vi "reward_behavior_timeout_10s_probes.vi"() -> ()   [LabVIEW 2019]
doc: "The myRIO Project template acquires acceleration data from the onboard accelerometer and displays the changes of acceleration values in a waveform chart."
uses:
  <vilib>/Analysis/Matrix/Datatypes/RealMatrix.ctl
  <vilib>/myRIO/Common/Instrument Driver Framework/myRIO v1.0/Encoder/typedefs/Encoder Signal Mode.ctl
  <vilib>/myRIO/Instrument Drivers/Onboard IO/Encoder/typedefs/Encoder Reference.ctl
  <vilib>/myRIO/Common/Instrument Driver Framework/Utilities/typedefs/myRIO Generic Hardware Reference.ctl
  <vilib>/myRIO/Common/Instrument Driver Framework/Utilities/typedefs/Hardware Version Enum.ctl
  <vilib>/myRIO/Common/Instrument Driver Framework/Utilities/typedefs/myRIO v1.0 Reference.ctl
  <vilib>/myRIO/Common/Instrument Driver Framework/Utilities/typedefs/Generic FPGA Reference.ctl
  <vilib>/myRIO/Common/Instrument Driver Framework/myRIO v1.0/Encoder/typedefs/Encoder Channels Enum.ctl
  <vilib>/myRIO/Common/Instrument Driver Framework/myRIO v1.0/Encoder/typedefs/Encoder Configuration v1.0.ctl
  <vilib>/userdefined/High Color/nirio_resource_hc.ctl
  <vilib>/myRIO/Instrument Drivers/Onboard IO/DIO/typedefs/DIO Reference.ctl
  <vilib>/myRIO/Common/Instrument Driver Framework/myRIO v1.0/DIO/typedefs/DIO Channels List.ctl
  <vilib>/myRIO/Common/Instrument Driver Framework/myRIO v1.0/DIO/typedefs/DIO Channels Enum.ctl
  <vilib>/myRIO/Common/Instrument Driver Framework/Utilities/vis/Is FPGA Ref Available.vi
  <vilib>/myRIO/Common/Instrument Driver Framework/myRIO v1.0/Encoder/vis/myRIO v1.1 Open Encoder.vi
  <vilib>/myRIO/Instrument Drivers/Onboard IO/Encoder/vis/Read.vi
  <vilib>/myRIO/Common/Instrument Driver Framework/myRIO v1.0/DIO/vis/myRIO v1.1 Open DIO.vi
  <vilib>/myRIO/Instrument Drivers/Onboard IO/DIO/vis/Write.vi
  <vilib>/myRIO/Instrument Drivers/Onboard IO/DIO/vis/Read.vi
  <vilib>/myRIO/Common/Instrument Driver Framework/Utilities/vis/Validate Channels.vi
  <vilib>/myRIO/Common/Instrument Driver Framework/myRIO v1.0/Encoder/vis/myRIO v1.0 Reserve Encoder.vi
  <vilib>/myRIO/Common/Instrument Driver Framework/myRIO v1.0/DIO/vis/myRIO v1.0 Reserve DIO.vi
  <vilib>/myRIO/Common/Instrument Driver Framework/myRIO v1.0/Encoder/vis/myRIO v1.0 Build MUX Configuration Encoder.vi
  <vilib>/myRIO/Common/Instrument Driver Framework/myRIO v1.0/Resource Manager/vis/myRIO v1.0 Reserve Channel List.vi
  <vilib>/myRIO/Common/Instrument Driver Framework/myRIO v1.0/DIO/vis/myRIO v1.0 Build MUX Configuration DIO.vi
  <vilib>/myRIO/Common/Instrument Driver Framework/myRIO v1.0/Resource Manager/vis/myRIO v1.0 Create Configuration List.vi
  <vilib>/myRIO/Common/Instrument Driver Framework/myRIO v1.0/Resource Manager/vis/myRIO v1.0 Reserve Channel.vi
  <vilib>/myRIO/Common/Instrument Driver Framework/myRIO v1.0/Resource Manager/vis/myRIO v1.0 Unreserve Channel.vi
  <vilib>/myRIO/Common/Instrument Driver Framework/myRIO v1.0/Resource Manager/vis/myRIO v1.0 Build Mutex Name.vi
  <vilib>/Utility/VariantDataType/GetNumericInfo.vi
  <vilib>/Utility/error.llb/Error Cluster From Error Code.vi
  <vilib>/myRIO/Common/Instrument Driver Framework/myRIO v1.0/myRIO v1.1 Open.vi
  <vilib>/myRIO/Common/Instrument Driver Framework/Utilities/vis/IO Manager.vi
  <vilib>/myRIO/Common/Instrument Driver Framework/Utilities/vis/Configuration Manager.vi
  <vilib>/myRIO/Common/Instrument Driver Framework/myRIO v1.0/Resource Manager/vis/myRIO v1.0 Configure IO.vi
  <vilib>/myRIO/Common/Instrument Driver Framework/myRIO v1.0/myRIO v1.0 Close.vi
  <vilib>/myRIO/Common/Instrument Driver Framework/myRIO v1.0/Encoder/vis/myRIO v1.0 Configure Encoder.vi
  <vilib>/myRIO/Common/Instrument Driver Framework/myRIO v1.0/Encoder/vis/myRIO v1.0 Read Encoder.vi
  <vilib>/myRIO/Common/Instrument Driver Framework/myRIO v1.0/DIO/vis/myRIO v1.0 Read DIO.vi
  <vilib>/myRIO/Common/Instrument Driver Framework/myRIO v1.0/DIO/vis/myRIO v1.0 Write DIO.vi
  <vilib>/myRIO/Express VI/Onboard IO/Encoder/Encoder Express VI.xnode
  <vilib>/myRIO/Instrument Drivers/Onboard IO/Encoder/vis/myRIO Encoder Open.xnode
  <vilib>/myRIO/Express VI/Onboard IO/DI/DI Express VI.xnode
  <vilib>/myRIO/Instrument Drivers/Onboard IO/DIO/vis/myRIO DIO Open.xnode
  <vilib>/myRIO/Express VI/Onboard IO/DO/DO Express VI.xnode
  <vilib>/myRIO/Instrument Drivers/Onboard IO/Encoder/Encoder.lvlib
  <vilib>/myRIO/Instrument Drivers/Onboard IO/DIO/DIO.lvlib
  <vilib>/Analysis/Matrix/NI_Matrix.lvlib
panel:
  in  "Give reward":bool
  out "Timings":dbl[](array[numeric])
  out "ISI":dbl
  out "ISI start time":dbl
  out "Time_out":bool=TRUE
  out "Time since lick":dbl
  out "Time of last lick":dbl
  out "Rewarded trials":dbl[](array[numeric])
  out "Rewards":u16
  out "Active Trial":bool
  out "Array temp2":T1
  out "Stimuli Loaded":bool
  out "Stim_ID":dbl[](array[numeric])
  out "Reward_mat":dbl[](array[numeric])
  out "Reward":bool=TRUE
  out "Frame clock":i32
  out "Licks":u32
  out "Lick":bool
  out "Time":dbl
  out "Stop":bool
  in  "Frames to collect":u32
  out "Overflow?":bool
  out "Counter Value":i32
  out "Velocity":dbl
  out "Velocity Plot":dbl[](graph)
  out "Velocity array":dbl[](array[numeric])
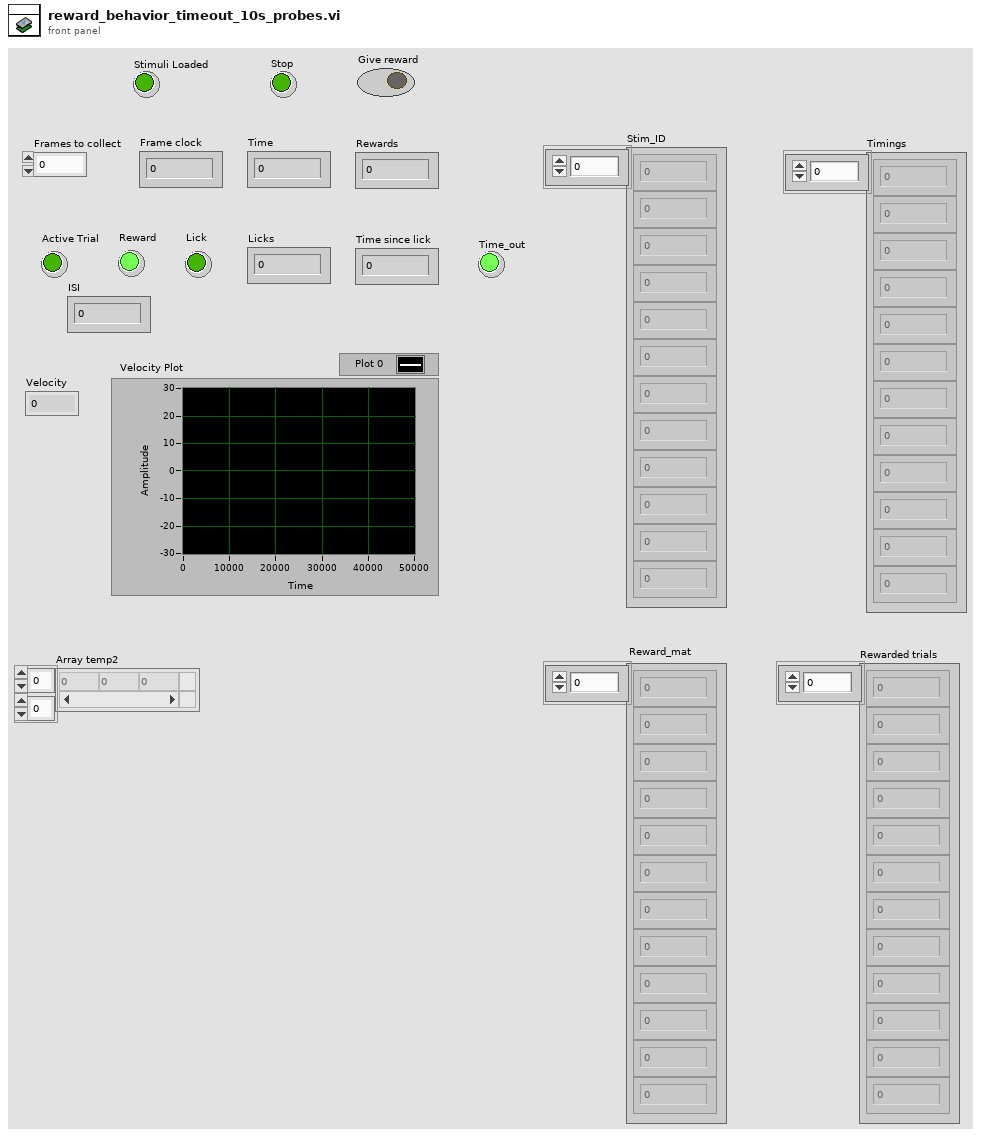
[diagram p1: front panel]
types:
  T1 = typedef "NI_Matrix.lvlib/RealMatrix.ctl" = dbl[][]
  T2 = typedef "Encoder.lvlib/Encoder Reference.ctl" = cluster{"myRIO Reference":T3, "Encoder Channels Enum":T7}
  T3 = typedef "myRIO Generic Hardware Reference.ctl" = cluster{"myRIO Model":T4, "myRIO Hardware Reference":T5}
  T4 = typedef "Hardware Version Enum.ctl" = enum16{"Unknown", "myRIO-1900", "myRIO-1950", "roboRIO", "NI ELVIS RIO CM", "ELVIS III"}
  T5 = typedef "myRIO v1.0 Reference.ctl" = cluster{"Generic FPGA Reference":T6, "Allow multiple opens":bool}
  T6 = typedef "Generic FPGA Reference.ctl" = refnum<k20>
  T7 = typedef "Encoder Channels Enum.ctl" = enum16{"Not Connected", "C/ENC0", "C/ENC1", "A/ENC", "A/ENC0", "A/ENC1", "A/ENC2", "A/ENC3", "A/ENC4", "A/ENC5", "A/ENC6", "A/ENC7", "A/ENC8", "A/ENC9", "B/ENC", "B/ENC0", "B/ENC1", "B/ENC2", "B/ENC3", "B/ENC4", "B/ENC5", "B/ENC6", "B/ENC7", "B/ENC8", "B/ENC9", "DIO/ENC0", "DIO/ENC1", "DIO/ENC2", "DIO/ENC3", "DIO/ENC4"}
  T8 = typedef "Encoder Signal Mode.ctl" = enum16{"Quadrature phase signal", "Step and direction signal"}
  T9 = typedef "nirio_resource_hc.ctl" = tag
  T10 = typedef "DIO.lvlib/DIO Reference.ctl" = cluster{"myRIO Reference":T3, "DIO Channels List":T11}
  T11 = typedef "DIO Channels List.ctl" = T12[]
  T12 = typedef "DIO Channels Enum.ctl" = enum16{"Not Connected", "C/DIO0", "C/DIO1", "C/DIO2", "C/DIO3", "C/DIO4", "C/DIO5", "C/DIO6", "C/DIO7", "A/DIO0", "A/DIO1", "A/DIO2", "A/DIO3", "A/DIO4", "A/DIO5", "A/DIO6", "A/DIO7", "A/DIO8", "A/DIO9", "A/DIO10", "A/DIO11", "A/DIO12", "A/DIO13", "A/DIO14", "A/DIO15", "A/DIO16", "A/DIO17", "A/DIO18", "A/DIO19", "B/DIO0", "B/DIO1", "B/DIO2", "B/DIO3", "B/DIO4", "B/DIO5", "B/DIO6", "B/DIO7", "B/DIO8", "B/DIO9", "B/DIO10", "B/DIO11", "B/DIO12", "B/DIO13", "B/DIO14", "B/DIO15", "B/DIO16", "B/DIO17", "B/DIO18", "B/DIO19", "LED0", "LED1", "LED2", "LED3", "Button0", "DIO/DIO0", "DIO/DIO1", "DIO/DIO2", "DIO/DIO3", "DIO/DIO4", "DIO/DIO5", "DIO/DIO6", "DIO/DIO7", "DIO/DIO8", "DIO/DIO9", "SPI/CS0", "SPI/CS1", "SPI/CS2", "SPI/CS3", "LED RADIO (Green)", "LED RADIO (Red)", "LED COMM (Green)", "LED COMM (Red)", "LED MODE (Green)", "LED MODE (Red)"}
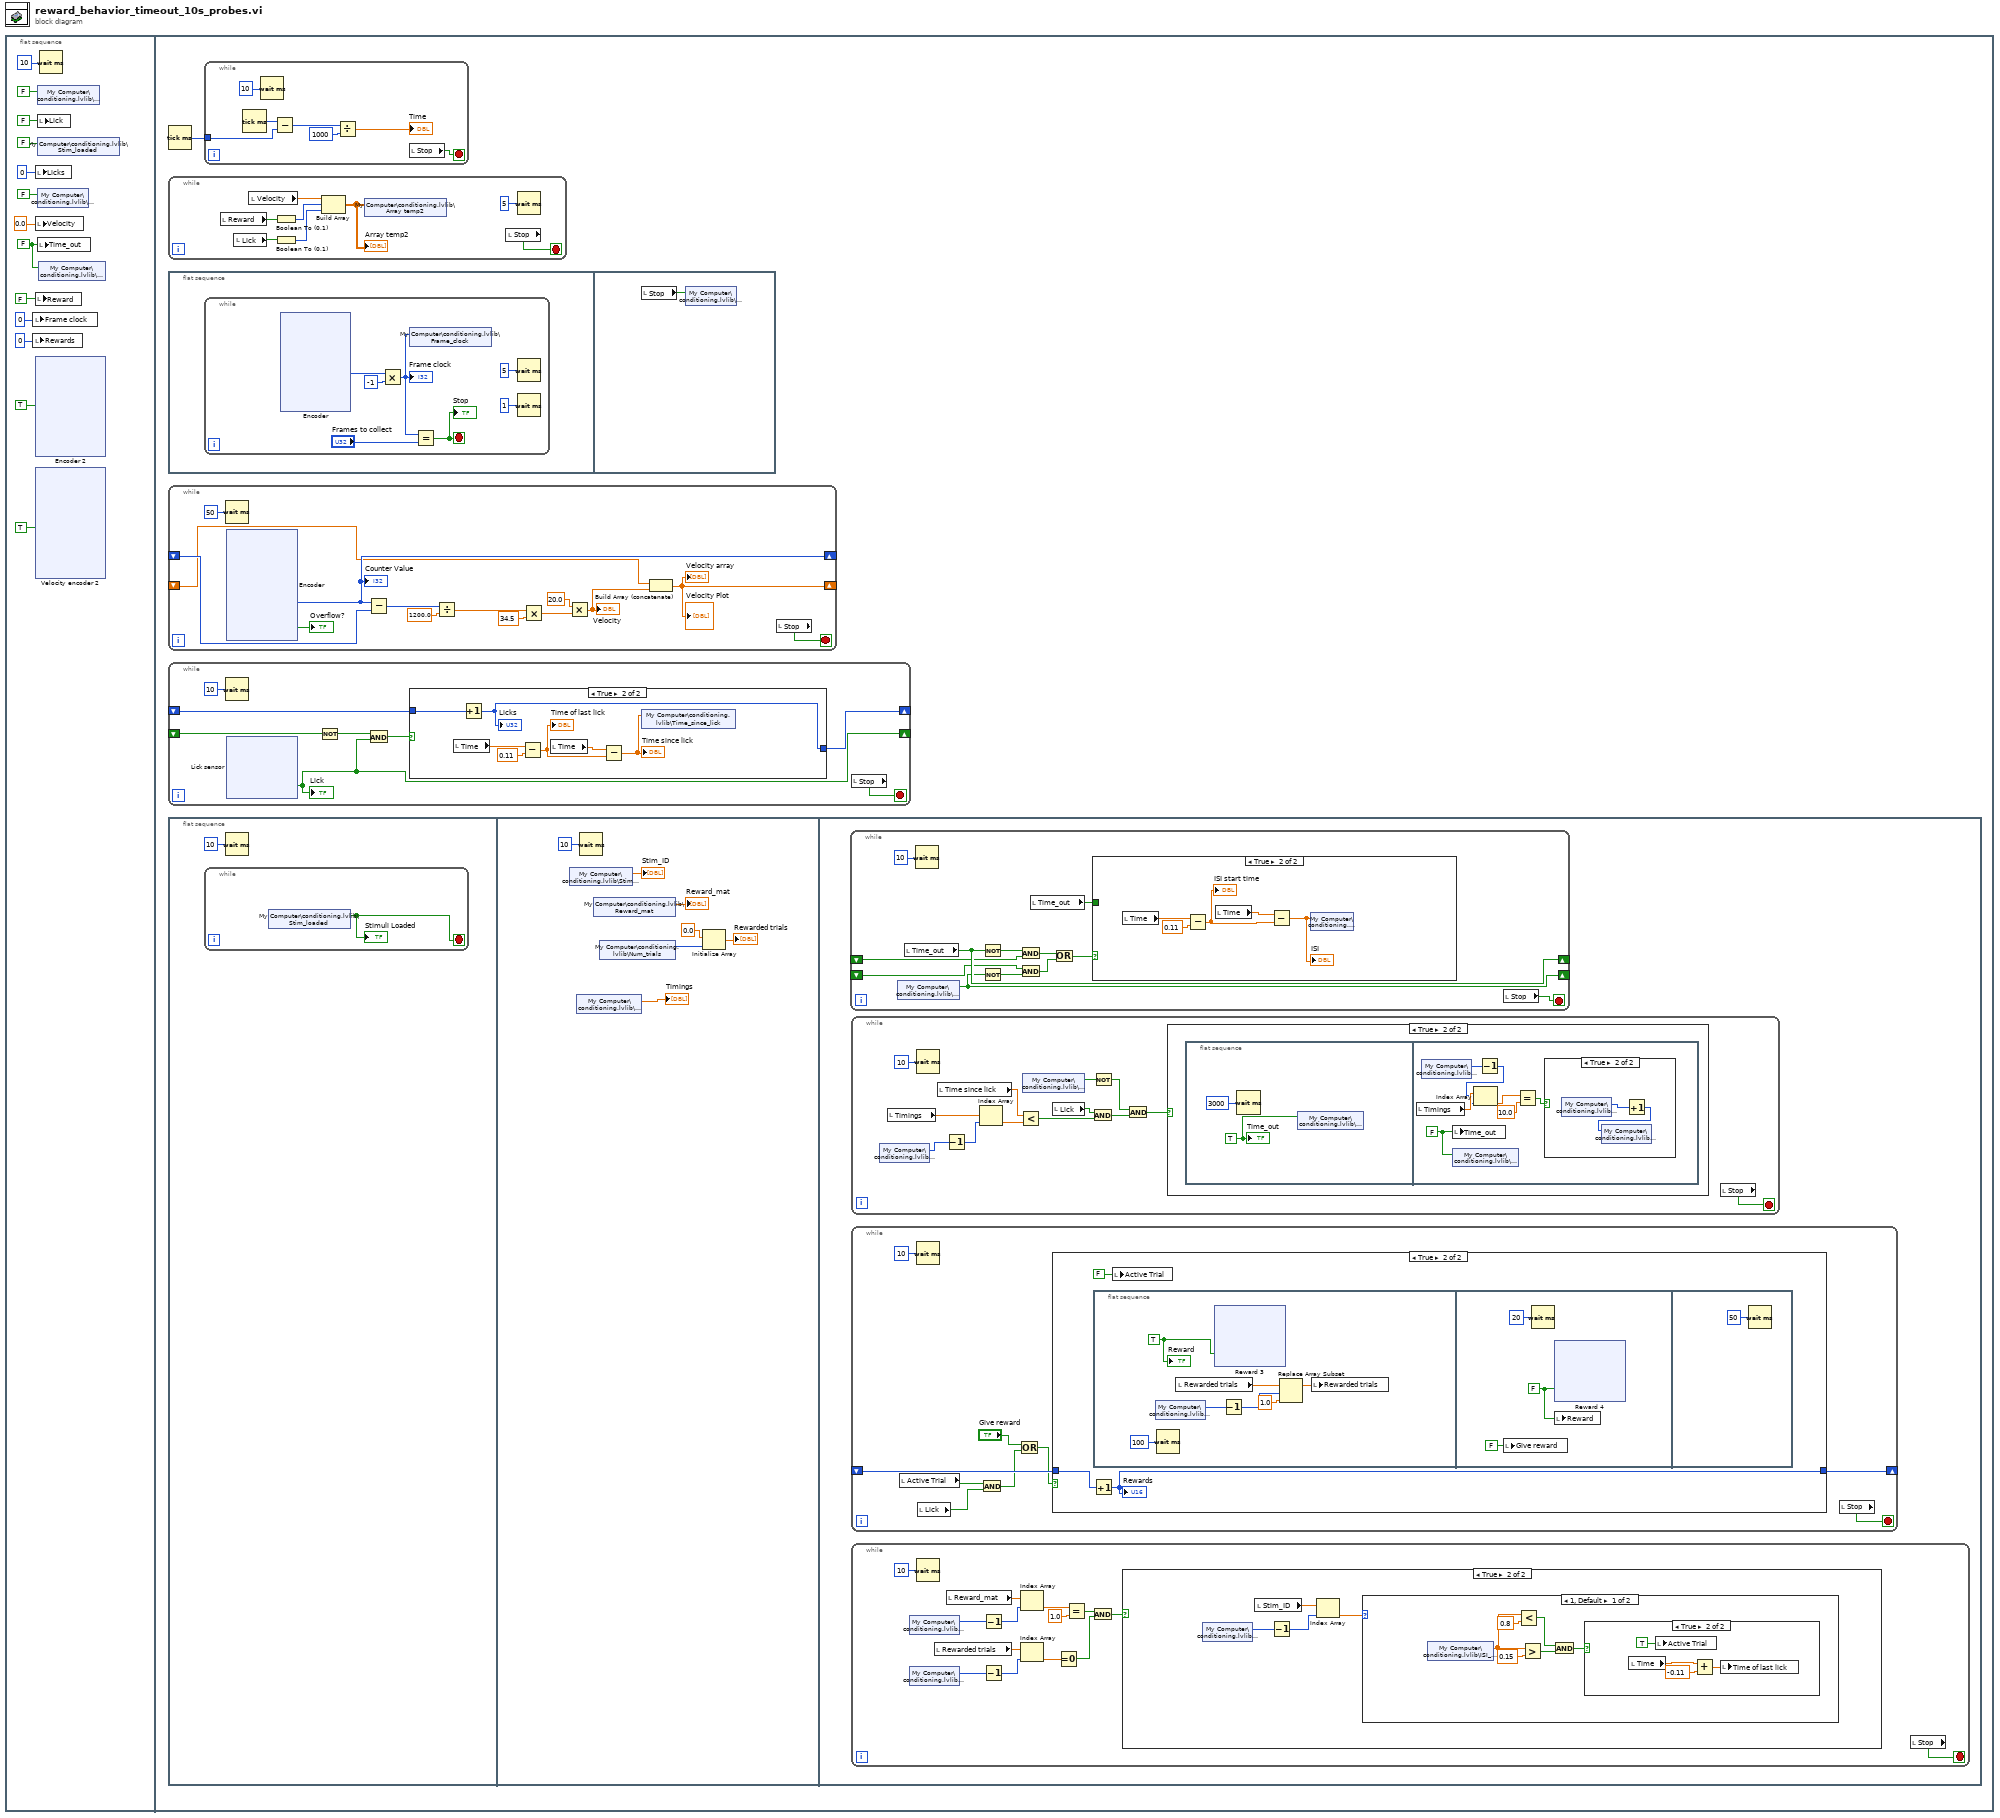
[diagram p0: block diagram]
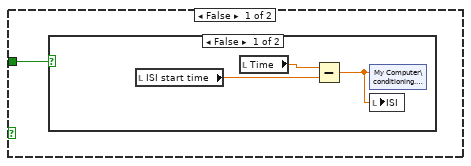
[diagram p4: hidden frame]
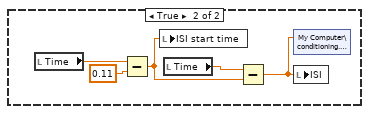
[diagram p5: hidden frame]
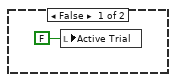
[diagram p6: hidden frame]
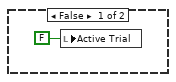
[diagram p7: hidden frame]
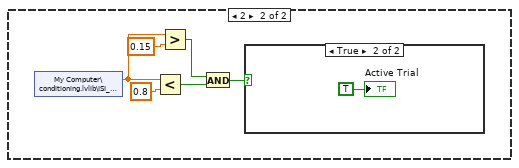
[diagram p8: hidden frame]
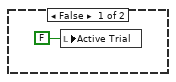
[diagram p9: hidden frame]
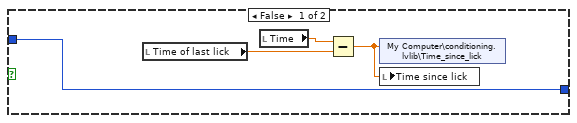
[diagram p11: hidden frame]
diagram:
  n1 = flat-sequence {
    frame #0 {
      w1 = FALSE ("Time_out")
      n2 = local write "Frame clock"(u32 0 ("Frames")) -> ()
      n3 = local write "Rewards"(u16 0 ("Rewards")) -> ()
      n4 = local write "Licks"(u32 0 ("Licks")) -> ()
      n5 = local write "Velocity"(0.0 ("Velocity")) -> ()
      n6 = local write "Reward"(FALSE ("Give reward")) -> ()
      n7 = xnode "Encoder 2"("Reset Counter"=TRUE) -> ()  [unwired: 1 in, 4 out]
      n8 = xnode "Velocity encoder 2"("Reset Counter"=TRUE) -> ()  [unwired: 1 in, 4 out]
      n9 = shared-variable "My Computer\\conditioning.lvlib\\Display"(FALSE ("Display")) -> ()  [unwired: 1 in, 1 out]
      n10 = local write "Lick"(FALSE ("Lick")) -> ()
      n11 = shared-variable "My Computer\\conditioning.lvlib\\Stim_loaded"(FALSE ("Stim_loaded")) -> ()  [unwired: 1 in, 1 out]
      n12 = shared-variable "My Computer\\conditioning.lvlib\\Stop"(FALSE ("Stop")) -> ()  [unwired: 1 in, 1 out]
      n13 = local write "Time_out"(w1) -> ()
      n14 = shared-variable "My Computer\\conditioning.lvlib\\Timeout"(w1) -> ()  [unwired: 1 in, 1 out]
      n15 = Wait (ms)(milliseconds to wait=u32 10) -> ()  [unwired: 1 out]
    }
    frame #1 {
      n16 = Tick Count (ms)() -> (millisecond timer value=w106:u32)
      n17 = while {
        stop <- w108 stop-if-true
        n18 = local read "Reward"() -> (w113:bool)
        n19 = local read "Lick"() -> (w114:bool)
        n20 = local read "Velocity"() -> (w112:dbl)
        n21 = Boolean To (0,1)(Boolean=w113) -> (0, 1=w111:i16)
        n22 = Boolean To (0,1)(Boolean=w114) -> (0, 1=w110:i16)
        n23 = Build Array(w112, w111, w110) -> (w107:T1)
        "Array temp2" <- w107
        n24 = shared-variable "My Computer\\conditioning.lvlib\\Array temp2"(w107) -> ()  [unwired: 1 in, 1 out]
        n25 = local read "Stop"() -> (w108:bool)
        n26 = Wait (ms)(milliseconds to wait=u32 5) -> ()  [unwired: 1 out]
      }
      n27 = flat-sequence {
        frame #0 {
          n28 = while {
            stop <- w307 stop-if-true
            n29 = xnode "Encoder"() -> ("Counter Value"=w311:i32)  [unwired: 2 in, 3 out]
            n30 = Multiply(x=w311, y=-1) -> (x*y=w306:i32)
            "Frame clock" <- w306
            n31 = shared-variable "My Computer\\conditioning.lvlib\\Frame_clock"(w306) -> ()  [unwired: 1 in, 1 out]
            n32 = Equal?(x=w306, y="Frames to collect") -> (x = y?=w307:bool)
            "Stop" <- w307
            n33 = Wait (ms)(milliseconds to wait=u32 5) -> ()  [unwired: 1 out]
            n34 = Wait (ms)(milliseconds to wait=u32 1) -> ()  [unwired: 1 out]
          }
        }
        frame #1 {
          n35 = local read "Stop"() -> (w359:bool)
          n36 = shared-variable "My Computer\\conditioning.lvlib\\Stop"(w359) -> ()  [unwired: 1 in, 1 out]
        }
      }
      n37 = while {
        shift-right: [w424] -> _
        shift-left: _ -> [w425]
        shift-right: [w416] -> _
        shift-left: _ -> [w415]
        stop <- w414 stop-if-true
        n38 = Wait (ms)(milliseconds to wait=u32 50) -> ()  [unwired: 1 out]
        n39 = xnode "Encoder"() -> ("Counter Value"=w424:i32, "Overflow?"=→"Overflow?":bool)  [unwired: 2 in, 2 out]
        "Counter Value" <- w424
        n40 = Subtract(x=w424, y=w425) -> (x-y=w417:i32)
        n41 = Divide(x=w417, y=1200.0 ("600")) -> (x/y=w422:dbl)
        n42 = Multiply(x=w422, y=34.5) -> (x*y=w420:dbl)
        n43 = Multiply(x=20.0, y=w420) -> (x*y=w418:dbl)
        "Velocity" <- w418
        n44 = Build Array (concatenate)(w415, w418) -> (w416:dbl[])
        "Velocity Plot" <- w416
        "Velocity array" <- w416
        n45 = local read "Stop"() -> (w414:bool)
      }
      n46 = while {
        shift-right: [w366] -> _
        shift-left: _ -> [w365]
        shift-right: [w360] -> _
        shift-left: _ -> [w363]
        stop <- w364 stop-if-true
        n47 = Wait (ms)(milliseconds to wait=u32 10) -> ()  [unwired: 1 out]
        n48 = xnode "Lick sensor"() -> ("C/DIO1 (DIO1)"=w360:bool)  [unwired: 1 in, 1 out]
        "Lick" <- w360
        n49 = Not(x=w363) -> (.not. x?=w362:bool)
        n50 = And(x=w362, y=w360) -> (x .and. y?=w361:bool)
        n51 = case shown="True" w361 {
          tunnel: [w371 w378] -> w366
          tunnel: w365 -> [w371 w377]
          frame False {
            n52 = local read "Time of last lick"() -> (w369:dbl)
            n53 = local read "Time"() -> (w370:dbl)
            n54 = Subtract(x=w370, y=w369) -> (x-y=w368:dbl)
            n55 = shared-variable "My Computer\\conditioning.lvlib\\Time_since_lick"(w368) -> ()  [unwired: 1 in, 1 out]
            n56 = local write "Time since lick"(w368) -> ()
          }
          frame True {
            n57 = local read "Time"() -> (w374:dbl)
            n58 = Increment(x=w377) -> (x+1=w378:u32)
            "Licks" <- w378
            n59 = Subtract(x=w374, y=0.11) -> (x-y=w372:dbl)
            "Time of last lick" <- w372
            n60 = local read "Time"() -> (w376:dbl)
            n61 = Subtract(x=w376, y=w372) -> (x-y=w375:dbl)
            "Time since lick" <- w375
            n62 = shared-variable "My Computer\\conditioning.lvlib\\Time_since_lick"(w375) -> ()  [unwired: 1 in, 1 out]
          }
        }
        n63 = local read "Stop"() -> (w364:bool)
      }
      n64 = flat-sequence {
        frame #0 {
          n65 = while {
            stop <- w116 stop-if-true
            n66 = shared-variable "My Computer\\conditioning.lvlib\\Stim_loaded"() -> (w116:bool)  [unwired: 1 in, 1 out]
            "Stimuli Loaded" <- w116
          }
          n67 = Wait (ms)(milliseconds to wait=u32 10) -> ()  [unwired: 1 out]
        }
        frame #1 {
          n68 = shared-variable "My Computer\\conditioning.lvlib\\Stim_ID"() -> (→"Stim_ID":dbl[])  [unwired: 1 in, 1 out]
          n69 = shared-variable "My Computer\\conditioning.lvlib\\Timings"() -> (→"Timings":dbl[])  [unwired: 1 in, 1 out]
          n70 = Wait (ms)(milliseconds to wait=u32 10) -> ()  [unwired: 1 out]
          n71 = shared-variable "My Computer\\conditioning.lvlib\\Reward_mat"() -> (→"Reward_mat":dbl[])  [unwired: 1 in, 1 out]
          n72 = shared-variable "My Computer\\conditioning.lvlib\\Num_trials"() -> (w120:u32)  [unwired: 1 in, 1 out]
          n73 = Initialize Array(0.0 ("element"), w120) -> (→"Rewarded trials":dbl[])
        }
        frame #2 {
          n74 = while {
            shift-right: [w158] -> _
            shift-left: _ -> [w156]
            shift-right: [w154] -> _
            shift-left: _ -> [w153]
            stop <- w159 stop-if-true
            n75 = shared-variable "My Computer\\conditioning.lvlib\\Display"() -> (w154:bool)  [unwired: 1 in, 1 out]
            n76 = local read "Time_out"() -> (w158:bool)
            n77 = Wait (ms)(milliseconds to wait=u32 10) -> ()  [unwired: 1 out]
            n78 = Not(x=w158) -> (.not. x?=w157:bool)
            n79 = Not(x=w154) -> (.not. x?=w152:bool)
            n80 = And(x=w157, y=w156) -> (x .and. y?=w151:bool)
            n81 = And(x=w153, y=w152) -> (x .and. y?=w150:bool)
            n82 = local read "Time_out"() -> (w155:bool)
            n83 = Or(x=w151, y=w150) -> (x .or. y?=w149:bool)
            n84 = case shown="True" w149 {
              tunnel: w155 -> [w160 _]
              frame False {
                n85 = case shown="False" w160 {
                  frame False {
                    n86 = local read "ISI start time"() -> (w163:dbl)
                    n87 = local read "Time"() -> (w162:dbl)
                    n88 = Subtract(x=w162, y=w163) -> (x-y=w161:dbl)
                    n89 = shared-variable "My Computer\\conditioning.lvlib\\ISI"(w161) -> ()  [unwired: 1 in, 1 out]
                    n90 = local write "ISI"(w161) -> ()
                  }
                  frame True {
                    n91 = local read "Time"() -> (w168:dbl)
                    n92 = Subtract(x=w168, y=0.11) -> (x-y=w165:dbl)
                    n93 = local write "ISI start time"(w165) -> ()
                    n94 = local read "Time"() -> (w166:dbl)
                    n95 = Subtract(x=w166, y=w165) -> (x-y=w164:dbl)
                    n96 = shared-variable "My Computer\\conditioning.lvlib\\ISI"(w164) -> ()  [unwired: 1 in, 1 out]
                    n97 = local write "ISI"(w164) -> ()
                  }
                }
              }
              frame True {
                n98 = local read "Time"() -> (w173:dbl)
                n99 = Subtract(x=w173, y=0.11) -> (x-y=w170:dbl)
                "ISI start time" <- w170
                n100 = local read "Time"() -> (w171:dbl)
                n101 = Subtract(x=w171, y=w170) -> (x-y=w169:dbl)
                "ISI" <- w169
                n102 = shared-variable "My Computer\\conditioning.lvlib\\ISI"(w169) -> ()  [unwired: 1 in, 1 out]
              }
            }
            n103 = local read "Stop"() -> (w159:bool)
          }
          n104 = while {
            stop <- w136 stop-if-true
            n105 = shared-variable "My Computer\\conditioning.lvlib\\Trial"() -> (w125:u32)  [unwired: 1 in, 1 out]
            n106 = local read "Timings"() -> (w127:dbl[])
            n107 = Wait (ms)(milliseconds to wait=u32 10) -> ()  [unwired: 1 out]
            n108 = local read "Time since lick"() -> (w135:dbl)
            n109 = Decrement(x=w125) -> (x-1=w124:u32)
            n110 = Index Array(array=w127, index=w124) -> (element=w126:dbl)
            n111 = Less?(x=w135, y=w126) -> (x < y?=w134:bool)
            n112 = shared-variable "My Computer\\conditioning.lvlib\\Display"() -> (w131:bool)  [unwired: 1 in, 1 out]
            n113 = local read "Lick"() -> (w133:bool)
            n114 = Not(x=w131) -> (.not. x?=w130:bool)
            n115 = And(x=w133, y=w134) -> (x .and. y?=w129:bool)
            n116 = And(x=w130, y=w129) -> (x .and. y?=w128:bool)
            n117 = case shown="True" w128 {
              frame False {
              }
              frame True {
                n118 = flat-sequence {
                  frame #0 {
                    w138 = TRUE
                    n119 = Wait (ms)(milliseconds to wait=u32 3000) -> ()  [unwired: 1 out]
                    n120 = shared-variable "My Computer\\conditioning.lvlib\\Timeout"(w138) -> ()  [unwired: 1 in, 1 out]
                    "Time_out" <- w138
                  }
                  frame #1 {
                    w145 = FALSE ("Timeout")
                    n121 = local read "Timings"() -> (w144:dbl[])
                    n122 = shared-variable "My Computer\\conditioning.lvlib\\Trial"() -> (w140:u32)  [unwired: 1 in, 1 out]
                    n123 = local write "Time_out"(w145) -> ()
                    n124 = shared-variable "My Computer\\conditioning.lvlib\\Timeout"(w145) -> ()  [unwired: 1 in, 1 out]
                    n125 = Decrement(x=w140) -> (x-1=w139:u32)
                    n126 = Index Array(array=w144, index=w139) -> (element=w142:dbl)
                    n127 = Equal?(x=w142, y=10.0) -> (x = y?=w143:bool)
                    n128 = case shown="True" w143 {
                      frame False {
                      }
                      frame True {
                        n129 = shared-variable "My Computer\\conditioning.lvlib\\Trial"() -> (w147:u32)  [unwired: 1 in, 1 out]
                        n130 = Increment(x=w147) -> (x+1=w146:u32)
                        n131 = shared-variable "My Computer\\conditioning.lvlib\\Trial"(w146) -> ()  [unwired: 1 in, 1 out]
                      }
                    }
                  }
                }
              }
            }
            n132 = local read "Stop"() -> (w136:bool)
          }
          n133 = while {
            shift-right: [w218] -> _
            shift-left: _ -> [w217]
            stop <- w220 stop-if-true
            n134 = local read "Active Trial"() -> (w216:bool)
            n135 = Wait (ms)(milliseconds to wait=u32 10) -> ()  [unwired: 1 out]
            n136 = local read "Lick"() -> (w212:bool)
            n137 = And(x=w216, y=w212) -> (x .and. y?=w215:bool)
            n138 = Or(x="Give reward", y=w215) -> (x .or. y?=w214:bool)
            n139 = case shown="True" w214 {
              tunnel: [w221 w224] -> w218
              tunnel: w217 -> [w221 w223]
              frame False {
              }
              frame True {
                n140 = Increment(x=w223) -> (x+1=w224:u16)
                "Rewards" <- w224
                n141 = flat-sequence {
                  frame #0 {
                    w230 = TRUE ("C/DIO0 (DIO0)")
                    n142 = shared-variable "My Computer\\conditioning.lvlib\\Trial"() -> (w229:u32)  [unwired: 1 in, 1 out]
                    n143 = Wait (ms)(milliseconds to wait=u32 100) -> ()  [unwired: 1 out]
                    n144 = local read "Rewarded trials"() -> (w227:dbl[])
                    n145 = xnode "Reward 3"("C/DIO0 (DIO0)"=w230) -> ()  [unwired: 1 in, 1 out]
                    n146 = Decrement(x=w229) -> (x-1=w228:u32)
                    n147 = Replace Array Subset(array=w227, new element=1.0 ("new element/subarray"), index=w228) -> (w225:dbl[])
                    n148 = local write "Rewarded trials"(w225) -> ()
                    "Reward" <- w230
                  }
                  frame #1 {
                    w269 = FALSE ("C/DIO0 (DIO0)")
                    n149 = local write "Give reward"(FALSE ("Give reward")) -> ()
                    n150 = Wait (ms)(milliseconds to wait=u32 20) -> ()  [unwired: 1 out]
                    n151 = xnode "Reward 4"("C/DIO0 (DIO0)"=w269) -> ()  [unwired: 1 in, 1 out]
                    n152 = local write "Reward"(w269) -> ()
                  }
                  frame #2 {
                    n153 = Wait (ms)(milliseconds to wait=u32 50) -> ()  [unwired: 1 out]
                  }
                }
                n154 = local write "Active Trial"(FALSE ("Active Trial")) -> ()
              }
            }
            n155 = local read "Stop"() -> (w220:bool)
          }
          n156 = while {
            stop <- w187 stop-if-true
            n157 = shared-variable "My Computer\\conditioning.lvlib\\Trial"() -> (w183:u32)  [unwired: 1 in, 1 out]
            n158 = shared-variable "My Computer\\conditioning.lvlib\\Trial"() -> (w179:u32)  [unwired: 1 in, 1 out]
            n159 = Wait (ms)(milliseconds to wait=u32 10) -> ()  [unwired: 1 out]
            n160 = local read "Rewarded trials"() -> (w180:dbl[])
            n161 = local read "Reward_mat"() -> (w182:dbl[])
            n162 = Decrement(x=w183) -> (x-1=w184:u32)
            n163 = Decrement(x=w179) -> (x-1=w178:u32)
            n164 = Index Array(array=w182, index=w184) -> (element=w185:dbl)
            n165 = Index Array(array=w180, index=w178) -> (element=w177:dbl)
            n166 = Equal To 0?(x=w177) -> (x = 0?=w176:bool)
            n167 = Equal?(x=w185, y=1.0) -> (x = y?=w175:bool)
            n168 = And(x=w175, y=w176) -> (x .and. y?=w174:bool)
            n169 = case shown="True" w174 {
              frame False {
                n170 = local write "Active Trial"(FALSE ("Active_trial")) -> ()
              }
              frame True {
                n171 = shared-variable "My Computer\\conditioning.lvlib\\Trial"() -> (w190:u32)  [unwired: 1 in, 1 out]
                n172 = local read "Stim_ID"() -> (w192:dbl[])
                n173 = Decrement(x=w190) -> (x-1=w191:u32)
                n174 = Index Array(array=w192, index=w191) -> (element=w189:dbl)
                n175 = case shown="1, Default" w189 {
                  frame 1, Default {
                    n176 = shared-variable "My Computer\\conditioning.lvlib\\ISI_Time"() -> (w197:dbl)  [unwired: 1 in, 1 out]
                    n177 = Less?(x=w197, y=0.8) -> (x < y?=w195:bool)
                    n178 = Greater?(x=w197, y=0.15) -> (0:w194:bool)
                    n179 = And(x=w195, y=w194) -> (x .and. y?=w193:bool)
                    n180 = case shown="True" w193 {
                      frame False {
                        n181 = local write "Active Trial"(FALSE ("Active Trial")) -> ()
                      }
                      frame True {
                        n182 = local read "Time"() -> (w202:dbl)
                        n183 = local write "Active Trial"(TRUE ("Active Trial")) -> ()
                        n184 = Add(x=w202, y=-0.11) -> (x+y=w200:dbl)
                        n185 = local write "Time of last lick"(w200) -> ()
                      }
                    }
                  }
                  frame 2 {
                    n186 = shared-variable "My Computer\\conditioning.lvlib\\ISI_Time"() -> (w208:dbl)  [unwired: 1 in, 1 out]
                    n187 = Less?(x=w208, y=0.8) -> (x < y?=w205:bool)
                    n188 = Greater?(x=w208, y=0.15) -> (0:w206:bool)
                    n189 = And(x=w206, y=w205) -> (x .and. y?=w204:bool)
                    n190 = case shown="True" w204 {
                      frame False {
                        n191 = local write "Active Trial"(FALSE ("Active Trial")) -> ()
                      }
                      frame True {
                        "Active Trial" <- TRUE ("Active Trial")
                      }
                    }
                  }
                }
              }
            }
            n192 = local read "Stop"() -> (w187:bool)
          }
        }
      }
      n193 = while {
        tunnel: w106 -> [w479]
        stop <- w477 stop-if-true
        n194 = Tick Count (ms)() -> (millisecond timer value=w480:u32)
        n195 = Wait (ms)(milliseconds to wait=u32 10) -> ()  [unwired: 1 out]
        n196 = Subtract(x=w480, y=w479) -> (x-y=w476:u32)
        n197 = Divide(x=w476, y=u32 1000) -> (x/y=→"Time":dbl)
        n198 = local read "Stop"() -> (w477:bool)
      }
    }
  }
